vi "666.vi"() -> ()   [LabVIEW 2013]
uses:
  <userlib>/KNR OS 3.0 LabVIEW Toolkit/Type Definition/Resource.ctl
  D:/WRO/WRO2016 LabVIEW2013/Program Files (x86)/National Instruments/LabVIEW 2015/user.lib/KNR OS 3.0 LabVIEW Toolkit/Type Definition/DC Motor Port.ctl
  Global 1.vi
  <userlib>/KNR OS 3.0 LabVIEW Toolkit/support SubVI/_Controls/Lego Port.ctl
panel:
  in  "STOP":bool
  out "Battery\nVoltage":dbl format="%#_13g"
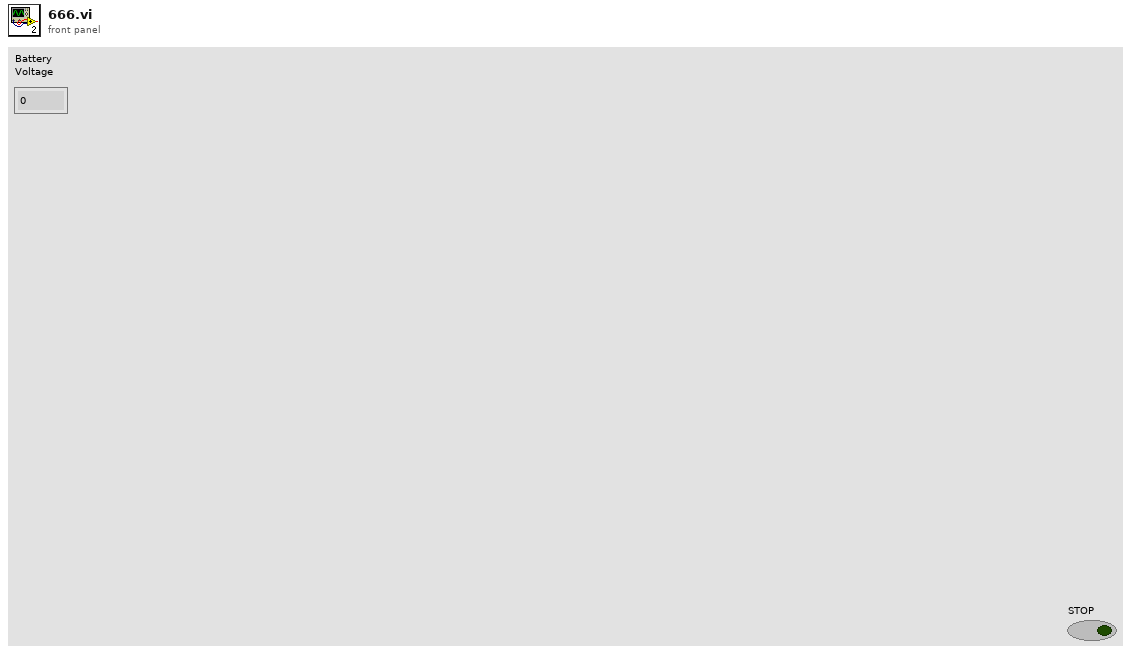
[diagram p1: front panel]
types:
  T1 = typedef "DC Motor Port.ctl" = u16
  T2 = typedef "Resource.ctl" = enum16{"KNRm_DDRC", "KNRm_DDDD", "KNRm_DDDR", "KNRm_DDDC", "KNR"}
  T3 = typedef "KNR3 Reference.ctl" = cluster{"FPGA Session":refnum<class "FPGA Interface Base.lvclass">, "Resource":T2}
  T4 = typedef "Lego Port.ctl" = enum8{"L1", "LS1", "LS3", "LS4", "LS2"}
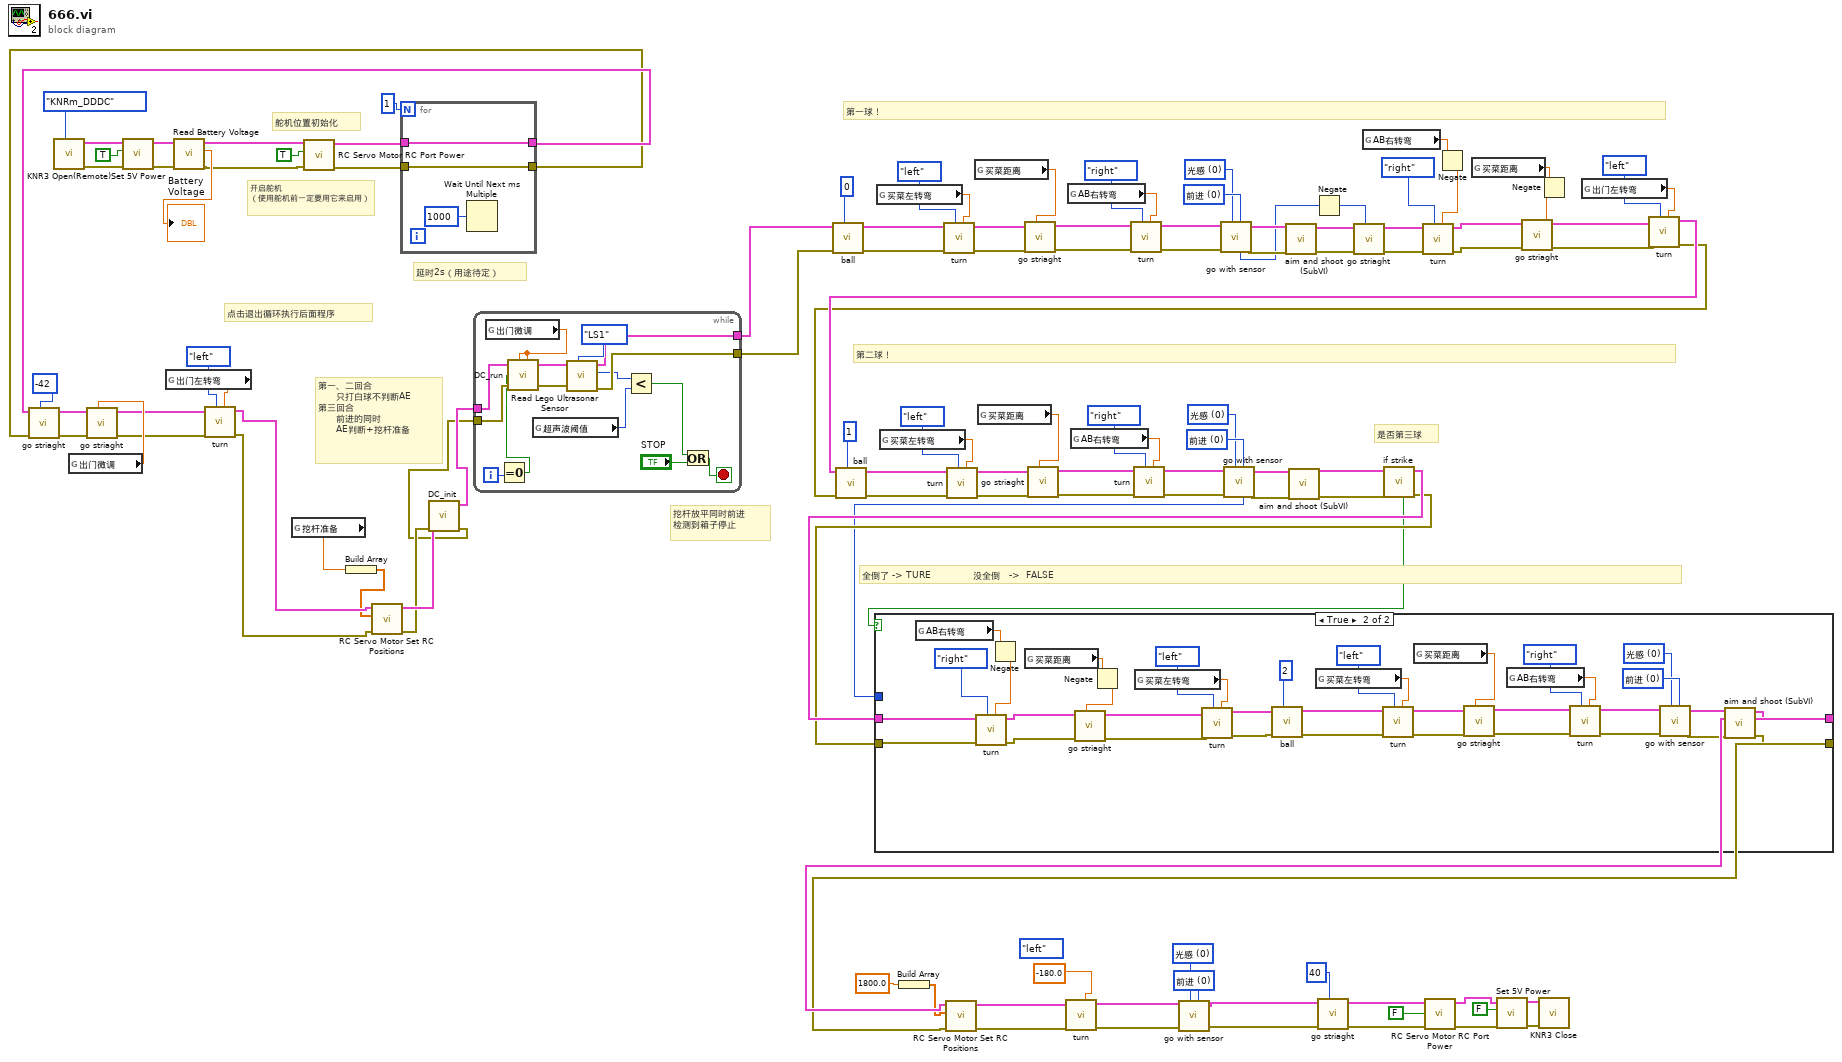
[diagram p0: block diagram]
diagram:
  w22 = T1 0 items=["前进", "后退"] ("方向")
  w23 = T1 0 items=["光感", "超声波"] ("传感器类型")
  (unwired) enum16{"right", "left"}."left"
  w56 = T1 0 items=["前进", "后退"] ("方向")
  w55 = T1 0 items=["光感", "超声波"] ("传感器类型")
  w89 = T1 0 items=["前进", "后退"] ("方向")
  w88 = T1 0 items=["光感", "超声波"] ("传感器类型")
  # "是否第三球"
  # "全倒了 -> TURE              没全倒   ->  FALSE"
  # "第二球！"
  # "第一球！"
  # "第一、二回合\n      只打白球不判断AE\n第三回合\n      前进的同时\n      AE判断+挖杆准备"
  # "挖杆放平同时前进\n检测到箱子停止"
  # "开启舵机\n（使用舵机前一定要用它来启用）"
  # "延时2s（用途待定）"
  # "舵机位置初始化"
  # "点击退出循环执行后面程序"
  n1 = call <userlib>:"KNR3 Open(Remote).vi"("Resource"=Resource."KNRm_DDDC") -> ("error out"=w114:errorcluster, "KNR out"=w115:T3)  [unwired: 9 in]
  n2 = global read "Global 1.vi" "出门微调"() -> (w103:dbl)
  n3 = call <userlib>:"Set 5V Power.vi"("error in (no error)"=w114, "5V Power(T)"=TRUE, "KNR in"=w115) -> ("error out"=w8:errorcluster, "KNR out"=w111:T3)  [unwired: 7 in]
  n4 = global read "Global 1.vi" "出门左转弯"() -> (w108:dbl)
  n5 = call <userlib>:"Read Battery Voltage.vi"("error in (no error)"=w8, "KNR in"=w111) -> ("error out"=w9:errorcluster, "Voltage"=→"Battery\nVoltage":dbl, "KNR out"=w10:T3)  [unwired: 7 in]
  n6 = global read "Global 1.vi" "挖杆准备"() -> (w32:dbl)
  n7 = call <userlib>:"RC Servo Motor RC Port Power.vi"("error in (no error)"=w9, "RC Power(F)"=TRUE, "KNR in"=w10) -> ("error out"=w11:errorcluster, "KNR out"=w12:T3)  [unwired: 7 in]
  n8 = Build Array(w32) -> (w31:dbl[])
  n9 = for {
    N: 1 -> [_]
    tunnel: w12 -> [w118]
    tunnel: w11 -> [w119]
    tunnel: [w119] -> w14
    tunnel: [w118] -> w15
    n10 = Wait Until Next ms Multiple(millisecond multiple=u32 1000) -> ()  [unwired: 1 out]
  }
  n11 = call "go striaght.vi"("距离"=-42, "error in (no error)"=w14, "KNR in"=w15) -> ("error out"=w104:errorcluster, "KNR out"=w105:T3)  [unwired: 7 in]
  n12 = call "go striaght.vi"("距离"=w103, "error in (no error)"=w104, "KNR in"=w105) -> ("error out"=w101:errorcluster, "KNR out"=w102:T3)  [unwired: 7 in]
  n13 = call "turn.vi"("Angle"=w108, "side"=enum16{"right", "left"}."left", "error in (no error)"=w101, "KNR in"=w102) -> ("error out"=w33:errorcluster, "KNR out"=w34:T3)  [unwired: 6 in]
  n14 = call <userlib>:"RC Servo Motor Set RC Positions.vi"("error in (no error)"=w33, "RC Pulse Width (1500 uS)"=w31, "KNR in"=w34) -> ("error out"=w3:errorcluster, "KNR out"=w4:T3)  [unwired: 7 in]
  n15 = call "DC_init.vi"("error in (no error)"=w3, "KNR in"=w4) -> ("error out"=w1:errorcluster, "KNR out"=w2:T3)  [unwired: 6 in, 2 out]
  n16 = while {
    tunnel: [w126] -> w6
    tunnel: [w125] -> w5
    tunnel: w2 -> [w133]
    tunnel: w1 -> [w132]
    i -> [w131]
    stop <- w120 stop-if-true
    n17 = global read "Global 1.vi" "出门微调"() -> (w134:dbl)
    n18 = Equal To 0?(x=w131) -> (x = 0?=w130:bool)
    n19 = call "DC_run.vi"("KNR in"=w133, "speed_1"=w134, "reinitialize? (F)"=w130, "error in (no error)"=w132, "speed_2"=w134) -> ("KNR out"=w128:T3, "error out"=w129:errorcluster)  [unwired: 1 in, 2 out]
    n20 = global read "Global 1.vi" "超声波阈值"() -> (w121:i32)
    n21 = call <userlib>:"Read Lego Ultrasonar Sensor.vi"("Port (LS1)"=Lego_Port."LS1", "error in (no error)"=w129, "KNR in"=w128) -> ("error out"=w125:errorcluster, "distance(cm)"=w122:u8, "KNR out"=w126:T3)  [unwired: 6 in]
    n22 = Less?(x=w122, y=w121) -> (x < y?=w124:bool)
    n23 = Or(x=w124, y="STOP") -> (x .or. y?=w120:bool)
  }
  n24 = call "ball.vi"("Numeric"=0, "error in (no error)"=w5, "KNR in"=w6) -> ("error out"=w98:errorcluster, "KNR out"=w99:T3)  [unwired: 7 in]
  n25 = global read "Global 1.vi" "买菜左转弯"() -> (w94:dbl)
  n26 = global read "Global 1.vi" "买菜左转弯"() -> (w61:dbl)
  n27 = Build Array(1800.0 ("element")) -> (w26:dbl[])
  n28 = call "turn.vi"("Angle"=w94, "side"=enum16{"right", "left"}."left", "error in (no error)"=w98, "KNR in"=w99) -> ("error out"=w96:errorcluster, "KNR out"=w97:T3)  [unwired: 6 in]
  n29 = global read "Global 1.vi" "买菜距离"() -> (w95:dbl)
  n30 = global read "Global 1.vi" "买菜距离"() -> (w62:dbl)
  n31 = call "go striaght.vi"("距离"=w95, "error in (no error)"=w96, "KNR in"=w97) -> ("error out"=w90:errorcluster, "KNR out"=w91:T3)  [unwired: 7 in]
  n32 = global read "Global 1.vi" "AB右转弯"() -> (w93:dbl)
  n33 = global read "Global 1.vi" "AB右转弯"() -> (w60:dbl)
  n34 = call "turn.vi"("Angle"=w93, "side"=enum16{"right", "left"}."right", "error in (no error)"=w90, "KNR in"=w91) -> ("error out"=w86:errorcluster, "KNR out"=w87:T3)  [unwired: 6 in]
  n35 = call "go with sensor.vi"("KNR in"=w87, "传感器类型"=w88, "error in (no error)"=w86, "方向"=w89) -> ("KNR out"=w85:T3, "offset"=w30:i32, "error out"=w84:errorcluster)  [unwired: 3 in]
  n36 = call "aim and shoot (SubVI).vi"("error in (no error)"=w84, "KNR in"=w85) -> ("error out"=w83:errorcluster, "KNR out"=w106:T3)  [unwired: 8 in]
  n37 = Negate(x=w30) -> (-x=w82:i32)
  n38 = call "go striaght.vi"("距离"=w82, "error in (no error)"=w83, "KNR in"=w106) -> ("error out"=w78:errorcluster, "KNR out"=w79:T3)  [unwired: 7 in]
  n39 = global read "Global 1.vi" "AB右转弯"() -> (w81:dbl)
  n40 = Negate(x=w81) -> (-x=w77:dbl)
  n41 = call "turn.vi"("Angle"=w77, "side"=enum16{"right", "left"}."right", "error in (no error)"=w78, "KNR in"=w79) -> ("error out"=w74:errorcluster, "KNR out"=w75:T3)  [unwired: 6 in]
  n42 = global read "Global 1.vi" "买菜距离"() -> (w76:dbl)
  n43 = Negate(x=w76) -> (-x=w73:dbl)
  n44 = call "go striaght.vi"("距离"=w73, "error in (no error)"=w74, "KNR in"=w75) -> ("error out"=w69:errorcluster, "KNR out"=w70:T3)  [unwired: 7 in]
  n45 = global read "Global 1.vi" "出门左转弯"() -> (w71:dbl)
  n46 = call "turn.vi"("Angle"=w71, "side"=enum16{"right", "left"}."left", "error in (no error)"=w69, "KNR in"=w70) -> ("error out"=w49:errorcluster, "KNR out"=w50:T3)  [unwired: 6 in]
  n47 = call "ball.vi"("Numeric"=1, "error in (no error)"=w49, "KNR in"=w50) -> ("error out"=w65:errorcluster, "KNR out"=w66:T3)  [unwired: 7 in]
  n48 = call "turn.vi"("Angle"=w61, "side"=enum16{"right", "left"}."left", "error in (no error)"=w65, "KNR in"=w66) -> ("error out"=w63:errorcluster, "KNR out"=w64:T3)  [unwired: 6 in]
  n49 = call "go striaght.vi"("距离"=w62, "error in (no error)"=w63, "KNR in"=w64) -> ("error out"=w57:errorcluster, "KNR out"=w58:T3)  [unwired: 7 in]
  n50 = call "turn.vi"("Angle"=w60, "side"=enum16{"right", "left"}."right", "error in (no error)"=w57, "KNR in"=w58) -> ("error out"=w53:errorcluster, "KNR out"=w54:T3)  [unwired: 6 in]
  n51 = call "go with sensor.vi"("KNR in"=w54, "传感器类型"=w55, "error in (no error)"=w53, "方向"=w56) -> ("KNR out"=w52:T3, "offset"=w16:i32, "error out"=w51:errorcluster)  [unwired: 3 in]
  n52 = call "aim and shoot (SubVI).vi"("error in (no error)"=w51, "KNR in"=w52) -> ("error out"=w47:errorcluster, "KNR out"=w48:T3)  [unwired: 8 in]
  n53 = call "if strike.vi"("error in (no error)"=w47, "KNR in"=w48) -> ("error out"=w45:errorcluster, "KNR out"=w46:T3, "is strike?"=w44:bool)  [unwired: 7 in]
  n54 = case shown="True" w44 {
    tunnel: w16 -> [_ _]
    tunnel: w46 -> [w136 w138]
    tunnel: w45 -> [w135 w137]
    tunnel: [w136 w140] -> w28
    tunnel: [w135 w139] -> w27
    frame False {
    }
    frame True {
      w148 = T1 0 items=["前进", "后退"] ("方向")
      w147 = T1 0 items=["光感", "超声波"] ("传感器类型")
      n55 = global read "Global 1.vi" "AB右转弯"() -> (w171:dbl)
      n56 = Negate(x=w171) -> (-x=w169:dbl)
      n57 = call "turn.vi"("Angle"=w169, "side"=enum16{"right", "left"}."right", "error in (no error)"=w137, "KNR in"=w138) -> ("error out"=w166:errorcluster, "KNR out"=w167:T3)  [unwired: 6 in]
      n58 = global read "Global 1.vi" "买菜距离"() -> (w168:dbl)
      n59 = Negate(x=w168) -> (-x=w165:dbl)
      n60 = call "go striaght.vi"("距离"=w165, "error in (no error)"=w166, "KNR in"=w167) -> ("error out"=w161:errorcluster, "KNR out"=w162:T3)  [unwired: 7 in]
      n61 = global read "Global 1.vi" "买菜左转弯"() -> (w163:dbl)
      n62 = call "turn.vi"("Angle"=w163, "side"=enum16{"right", "left"}."left", "error in (no error)"=w161, "KNR in"=w162) -> ("error out"=w141:errorcluster, "KNR out"=w142:T3)  [unwired: 6 in]
      n63 = call "ball.vi"("Numeric"=2, "error in (no error)"=w141, "KNR in"=w142) -> ("error out"=w157:errorcluster, "KNR out"=w158:T3)  [unwired: 7 in]
      n64 = global read "Global 1.vi" "买菜左转弯"() -> (w153:dbl)
      n65 = call "turn.vi"("Angle"=w153, "side"=enum16{"right", "left"}."left", "error in (no error)"=w157, "KNR in"=w158) -> ("error out"=w155:errorcluster, "KNR out"=w156:T3)  [unwired: 6 in]
      n66 = global read "Global 1.vi" "买菜距离"() -> (w154:dbl)
      n67 = call "go striaght.vi"("距离"=w154, "error in (no error)"=w155, "KNR in"=w156) -> ("error out"=w149:errorcluster, "KNR out"=w150:T3)  [unwired: 7 in]
      n68 = global read "Global 1.vi" "AB右转弯"() -> (w152:dbl)
      n69 = call "turn.vi"("Angle"=w152, "side"=enum16{"right", "left"}."right", "error in (no error)"=w149, "KNR in"=w150) -> ("error out"=w145:errorcluster, "KNR out"=w146:T3)  [unwired: 6 in]
      n70 = call "go with sensor.vi"("KNR in"=w146, "传感器类型"=w147, "error in (no error)"=w145, "方向"=w148) -> ("KNR out"=w144:T3, "error out"=w143:errorcluster)  [unwired: 3 in, 1 out]
      n71 = call "aim and shoot (SubVI).vi"("error in (no error)"=w143, "KNR in"=w144) -> ("error out"=w139:errorcluster, "KNR out"=w140:T3)  [unwired: 8 in]
    }
  }
  n72 = call <userlib>:"RC Servo Motor Set RC Positions.vi"("error in (no error)"=w27, "RC Pulse Width (1500 uS)"=w26, "KNR in"=w28) -> ("error out"=w24:errorcluster, "KNR out"=w25:T3)  [unwired: 7 in]
  n73 = call "turn.vi"("Angle"=-180.0, "error in (no error)"=w24, "KNR in"=w25) -> ("error out"=w20:errorcluster, "KNR out"=w21:T3)  [unwired: 7 in]
  n74 = call "go with sensor.vi"("KNR in"=w21, "传感器类型"=w23, "error in (no error)"=w20, "方向"=w22) -> ("KNR out"=w19:T3, "error out"=w18:errorcluster)  [unwired: 3 in, 1 out]
  n75 = call "go striaght.vi"("距离"=40, "error in (no error)"=w18, "KNR in"=w19) -> ("error out"=w35:errorcluster, "KNR out"=w36:T3)  [unwired: 7 in]
  n76 = call <userlib>:"RC Servo Motor RC Port Power.vi"("error in (no error)"=w35, "RC Power(F)"=FALSE, "KNR in"=w36) -> ("error out"=w37:errorcluster, "KNR out"=w38:T3)  [unwired: 7 in]
  n77 = call <userlib>:"Set 5V Power.vi"("error in (no error)"=w37, "5V Power(T)"=FALSE, "KNR in"=w38) -> ("error out"=w41:errorcluster, "KNR out"=w40:T3)  [unwired: 7 in]
  n78 = call <userlib>:"KNR3 Close.vi"("error in (no error)"=w41, "KNR in"=w40) -> ()  [unwired: 9 in, 1 out]
